vi "Stop on Stop or Error.vi"(8 "error in (no error)":errorcluster) -> (0 "error out":errorcluster, 3 "Boolean":bool)   [LabVIEW 2024]
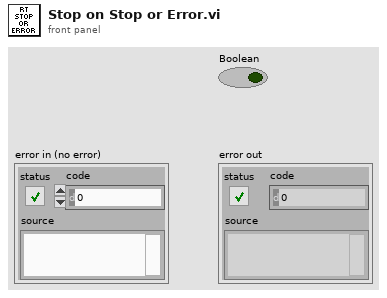
[diagram p1: front panel]
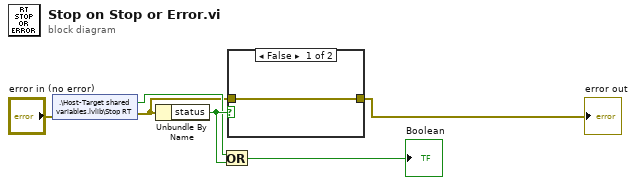
[diagram p0: block diagram]
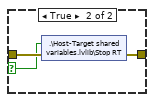
[diagram p2: hidden frame]
diagram:
  n1 = shared-variable ".\\Host-Target shared variables.lvlib\\Stop RT"(error in="error in (no error)") -> (w4:bool, error out=w3:errorcluster)
  n2 = Unbundle By Name(w3) -> ("status"=w6:bool)
  n3 = Or(x=w4, y=w6) -> (x .or. y?=→"Boolean":bool)
  n4 = case shown="False" w6 {
    selector: w6 -> [_ w8]
    tunnel: [w7 w10] -> w1
    tunnel: w3 -> [w7 w9]
    frame False {
    }
    frame True {
      n5 = shared-variable ".\\Host-Target shared variables.lvlib\\Stop RT"(w8, error in=w9) -> (error out=w10:errorcluster)
    }
  }
  "error out" <- w1
